vi "sensor cmd user calibration data.vi"(10 "sensor_comp":T1, 11 "dev_handle":u32) -> (1 "function return":i32, 2 "sensor_comp out":T1, 3 "dev_handle out":u32)   [LabVIEW 2019, in "apdm.lvlib"]
doc: "APDM_EXPORT int apdm_sensor_cmd_user_calibration_data(apdm_device_handle_t dev_handle, apdm_sensor_compensation_t *sensor_comp);"
uses:
  apdm.lvlib
  Lee Lab/CP FES Walking 2018/Code/Working/LabVIEW/apdm.dll
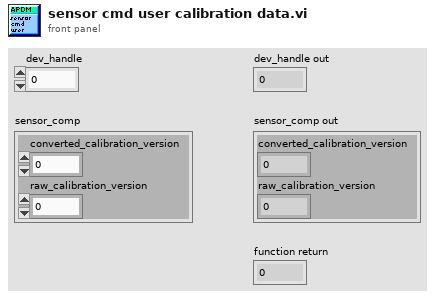
[diagram p1: front panel]
types:
  T1 = cluster{"converted_calibration_version":u32, "raw_calibration_version":u32}
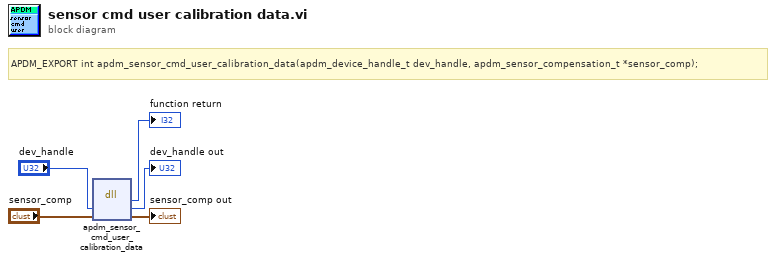
[diagram p0: block diagram]
diagram:
  # "APDM_EXPORT int apdm_sensor_cmd_user_calibration_data(apdm_device_handle_t dev_handle, apdm_sensor_compensation_t *sensor_comp);"
  n1 = dll-call lib="C:/Users/jfalesi/Dropbox/Lee Lab/CP FES Walking 2018/Code/Working/LabVIEW/apdm.*" fn="apdm_sensor_cmd_user_calibration_data"("dev_handle"="dev_handle", "sensor_comp"="sensor_comp") -> (→"function return":i32, "dev_handle"=→"dev_handle out":u32, "sensor_comp"=→"sensor_comp out":T1)  [unwired: 3 in, 2 out]
